vi "converte_P+T_to_massaespecífica.vi"() -> ()   [LabVIEW 2019]
panel:
  out "Max_vap":dbl
  out "Min_vap":dbl
  out "Min_liq":dbl
  out "Max_liq":dbl
  in  "Press [bar]":dbl[](array[numeric])
  in  "Temp [ºC]":dbl[](array[numeric])
  in  "error in (no error)":errorcluster
  in  "Refrigerant File":string="R134a.fld"
  in  "Refprop installation directory":path=path "c:/arquivos de programas/NIST/refprop7"
  out "error out":errorcluster
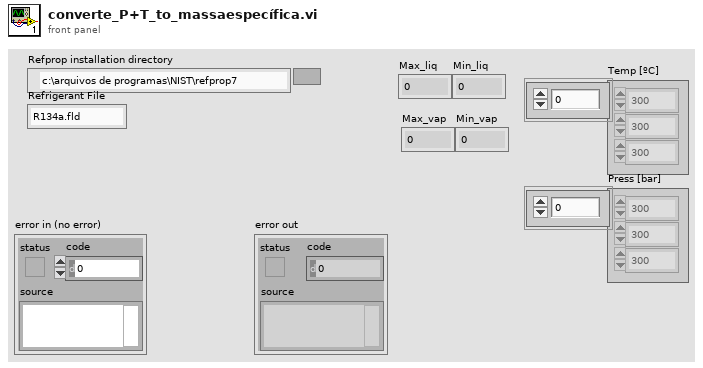
[diagram p1: front panel]
types:
  T1 = cluster{"Overall molar density [mol/l] (d)":dbl, "Molar density of the liquid phase [mol/l] (Dl)":dbl, "Molar density of the vapor phase [mol/l] (Dv)":dbl, "Liquid composition (xliq)":dbl[], "Vapor composition (xvap)":dbl[], "Vapor quality on a molar basis (q)":dbl, "Internal energy [J/mol] (e)":dbl, "Enthalpy [J/mol] (h)":dbl, "Entropy [J/(mol.K)] (s)":dbl, "Isochoric heat capacity [J/(mol.K)] (Cv)":dbl, "Isobaric heat capacity [J/(mol.K)] (Cp)":dbl, "Speed of sound [m/s] (w)":dbl}
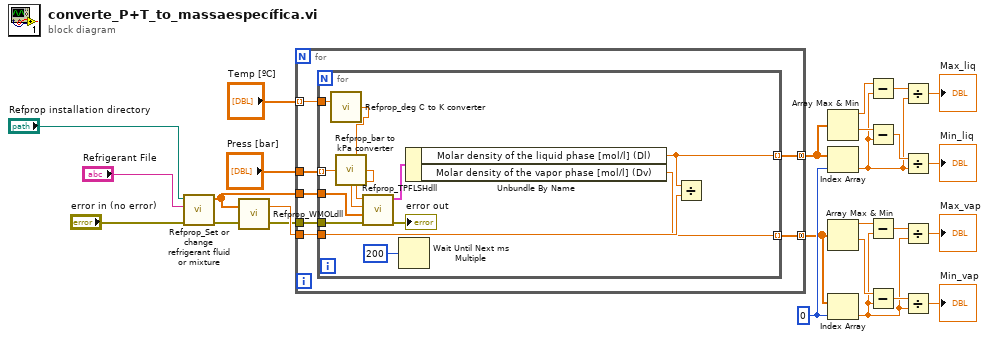
[diagram p0: block diagram]
diagram:
  w17 = 0 ("index")
  n1 = call "Refprop_Set or change refrigerant fluid or mixture.vi"("error in (no error)"="error in (no error)", "Refrigerant File (R134a.fld)"="Refrigerant File", "Refprop installation directory"="Refprop installation directory") -> ("error out"=w24:errorcluster, "Component molar fractions"=w23:dbl[])  [unwired: 7 in]
  n2 = call "Refprop_WMOLdll.vi"("error in (no error)"=w24, "Component molar fractions"=w23) -> ("error out"=w25:errorcluster, "Molar mass [g/mol]"=w26:dbl)
  n3 = for {
    tunnel: w26 -> [w33]
    tunnel: w25 -> [w32]
    tunnel: w23 -> [w31]
    tunnel: "Temp [ºC]" -> [w30] mode=indexing
    tunnel: "Press [bar]" -> [w29]
    tunnel: [w28] -> w16 mode=concatenating
    tunnel: [w27] -> w2 mode=concatenating
    n4 = for {
      tunnel: w31 -> [w40]
      tunnel: w33 -> [w44]
      tunnel: w32 -> [w41]
      tunnel: w30 -> [w34]
      tunnel: w29 -> [w36] mode=indexing
      tunnel: [w39] -> w28 mode=indexing
      tunnel: [w38] -> w27 mode=indexing
      n5 = call "Refprop_deg C to K converter.vi"("temperature [ºC]"=w34) -> ("temperature [K]"=w35:dbl)  [unwired: 4 in]
      n6 = call "Refprop_bar to kPa converter.vi"("pressure [bar]"=w36) -> ("pressure [kPa]"=w37:dbl)  [unwired: 4 in]
      n7 = call "Refprop_TPFLSHdll.vi"("error in (no error)"=w41, "Component molar fractions"=w40, "Pressure [kPa]"=w37, "Temperature [K]"=w35) -> ("error out"=→"error out":errorcluster, "TPFLSH output cluster"=w45:T1)  [unwired: 3 in, 1 out]
      n8 = Wait Until Next ms Multiple(millisecond multiple=u32 200) -> ()  [unwired: 1 out]
      n9 = Unbundle By Name(w45) -> ("Molar density of the liquid phase [mol/l] (Dl)"=w39:dbl, "Molar density of the vapor phase [mol/l] (Dv)"=w38:dbl)
      n10 = Divide(x=w39, y=w44) -> ()  [unwired: 1 out]
    }
  }
  n11 = Array Max & Min(array=w16) -> (max value=w15:dbl, min value=w14:dbl)  [unwired: 2 out]
  n12 = Index Array(array=w16, index=w17) -> (element=w11:dbl)
  n13 = Array Max & Min(array=w2) -> (max value=w3:dbl, min value=w4:dbl)  [unwired: 2 out]
  n14 = Index Array(array=w2, index=w17) -> (element=w1:dbl)
  n15 = Subtract(x=w15, y=w11) -> (x-y=w13:dbl)
  n16 = Subtract(x=w14, y=w11) -> (x-y=w12:dbl)
  n17 = Subtract(x=w3, y=w1) -> (x-y=w5:dbl)
  n18 = Subtract(x=w4, y=w1) -> (x-y=w6:dbl)
  n19 = Divide(x=w13, y=w11) -> (x/y=→"Max_liq":dbl)
  n20 = Divide(x=w12, y=w11) -> (x/y=→"Min_liq":dbl)
  n21 = Divide(x=w5, y=w1) -> (x/y=→"Max_vap":dbl)
  n22 = Divide(x=w6, y=w1) -> (x/y=→"Min_vap":dbl)
